vi "matlab-script-test.vi"   [LabVIEW 2018]
uses:
  <vilib>/measure/NI_MABase.lvlib
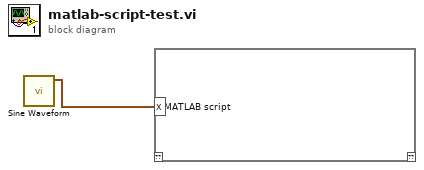
[diagram p0: block diagram]
diagram:
  n1 = call <vilib>:"Sine Waveform.vi"() -> ("signal out"=w1:waveform(dbl))  [unwired: 10 in, 1 out]
  n2 = script code="MATLAB script"("X"=w1) -> ()  [unwired: 1 in, 1 out]
